vi "Audio.Play_Record.vi"(5 "volume":dbl=40.0 format="%#_13g", 6 "Record Device ID":u32, 7 "Play Device ID":u32=1, 8 "error in (no error)":errorcluster, 9 "RcdPostTime":dbl=0.05 format="%#_13g", 10 "RcdPreTime":dbl=0.05 format="%#_13g", 11 "Play Wvfrm":waveform(dbl)[](array[waveform])) -> (0 "Error Out":errorcluster, 2 "PlayDur(s)":dbl=1.0 format="%.2p", 3 "Rcd Wvfrm":waveform(dbl)[](array[waveform]))   [LabVIEW 2018]
uses:
  <vilib>/sound2/lvsound2.llb/Sampling Mode.ctl
  <vilib>/sound2/lvsound2.llb/Sound Data Format.ctl
  Utils/Errors/Error.Error Code List.ctl
  <vilib>/sound2/lvsound2.llb/Sound Output Set Volume (Single).vi
  <vilib>/sound2/lvsound2.llb/Sound Input Read (DBL).vi
  <vilib>/sound2/lvsound2.llb/Sound Output Write (DBL).vi
  <vilib>/KATE/Time/Time Utils.lvlib
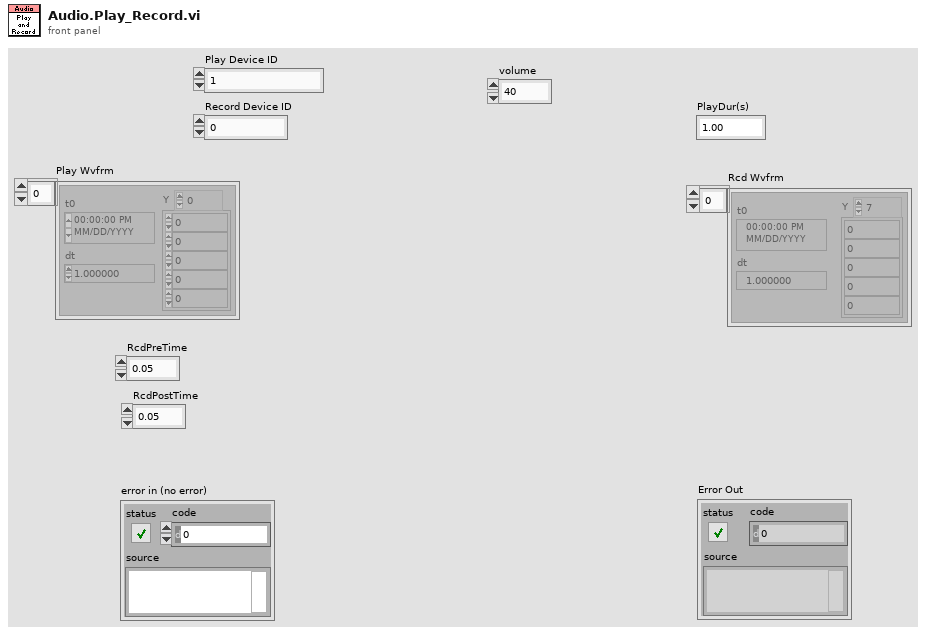
[diagram p1: front panel]
types:
  T1 = typedef "Sound Data Format.ctl" = cluster{"sample rate (S/s)":dbl, "number of channels":i32, "bits per sample":i32}
  T2 = typedef "Error.Error Code List.ctl" = i32
  T3 = typedef "Sampling Mode.ctl" = i32
  T4 = typedef "Sound Output Task ID.ctl" = u32
  T5 = typedef "Sound Input Task ID.ctl" = u32
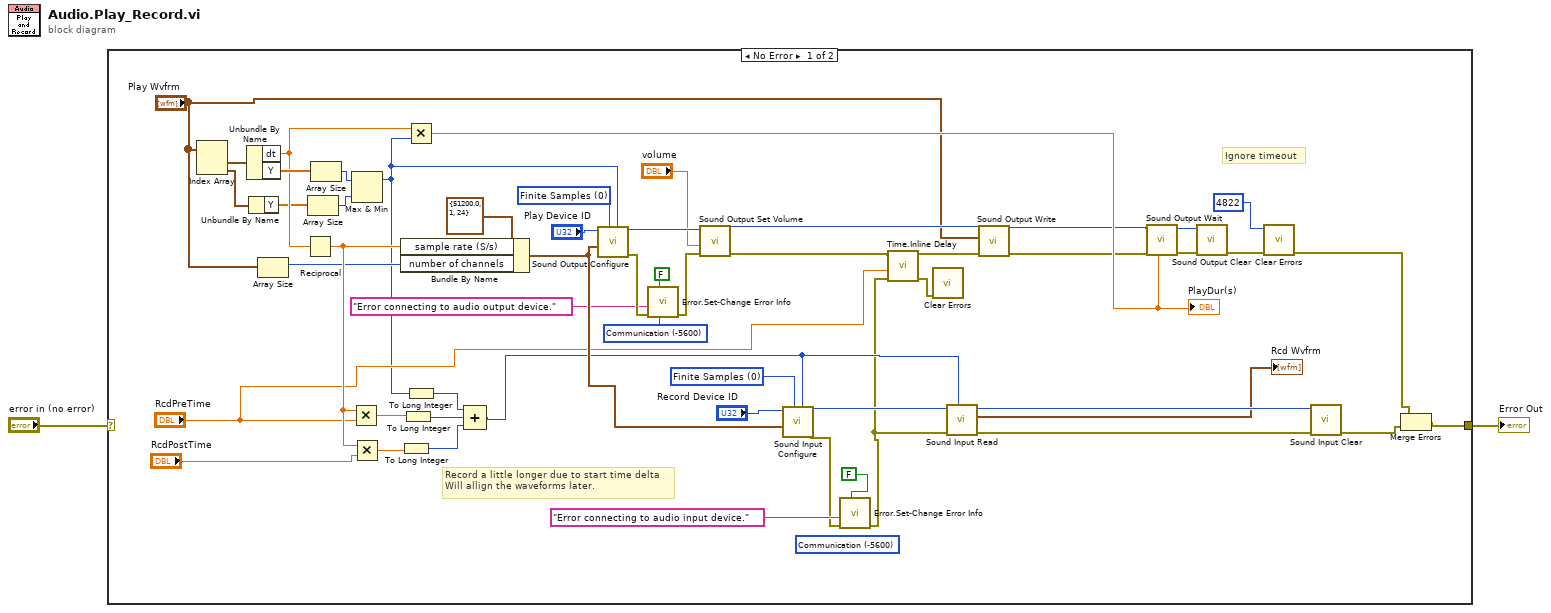
[diagram p0: block diagram]
diagram:
  n1 = case shown="No Error" "error in (no error)" {
    selector: "error in (no error)" -> [_ w57]
    tunnel: [w37 w57] -> w2
    frame No Error {
      (unwired) T2 -5600 items=["No Error"=0, "Abort"=-2, "Misc"=-5000, "Fixture Error"=-5100, "File IO - General"=-5200, "FIle IO - Config Error"=-5201, "Instrument - General"=-5300, "Instrument - Serial Com"=-5301, "Instrument - Camera"=-5302, "Instrument - PS"=-5303, "Instrument - Oscilloscope"=-5304, "Instrument - Function Gen"=-5305, "Instrument - Load"=-5306, "Instrument - Meter"=-5307, "Instrument - Power Control"=-5308, "Instrument - Motion"=-5309, "Instrument - RF"=-5310, "System Exe"=-5400, "Image Processing"=-5500, "Communication"=-5600, "Script - Syntax Error"=-6000, "Script - Invalid Name or Param"=-6100, "Script - Timeout"=-6200, "Invalid Data"=-6300, "FW Update Error"=-6500] ("Std Code")
      w34 = T2 -5600 items=["No Error"=0, "Abort"=-2, "Misc"=-5000, "Fixture Error"=-5100, "File IO - General"=-5200, "FIle IO - Config Error"=-5201, "Instrument - General"=-5300, "Instrument - Serial Com"=-5301, "Instrument - Camera"=-5302, "Instrument - PS"=-5303, "Instrument - Oscilloscope"=-5304, "Instrument - Function Gen"=-5305, "Instrument - Load"=-5306, "Instrument - Meter"=-5307, "Instrument - Power Control"=-5308, "Instrument - Motion"=-5309, "Instrument - RF"=-5310, "System Exe"=-5400, "Image Processing"=-5500, "Communication"=-5600, "Script - Syntax Error"=-6000, "Script - Invalid Name or Param"=-6100, "Script - Timeout"=-6200, "Invalid Data"=-6300, "FW Update Error"=-6500] ("Std Code")
      w51 = T3 0 items=["Finite Samples", "Continuous Samples"] ("sample mode")
      w53 = T3 0 items=["Finite Samples", "Continuous Samples"] ("sample mode")
      # "Ignore timeout"
      # "Record a little longer due to start time delta\nWill allign the waveforms later."
      n2 = Index Array(array="Play Wvfrm") -> (element #1=w28:waveform(dbl), element #2=w7:waveform(dbl))  [unwired: 2 in]
      n3 = Unbundle By Name(w28) -> ("dt"=w26:dbl, "Y"=w48:dbl[])
      n4 = Unbundle By Name(w7) -> ("Y"=w6:dbl[])
      n5 = Array Size(array="Play Wvfrm") -> (size(s)=w8:i32)
      n6 = Reciprocal(x=w26) -> (1/x=w25:dbl)
      n7 = Array Size(array=w6) -> (size(s)=w4:i32)
      n8 = Array Size(array=w48) -> (size(s)=w5:i32)
      n9 = Multiply(x=w25, y="RcdPreTime") -> (x*y=w47:dbl)
      n10 = Max & Min(x=w5, y=w4) -> (max(x,y)=w3:i32)  [unwired: 1 out]
      n11 = Multiply(x=w25, y="RcdPostTime") -> (x*y=w21:dbl)
      n12 = Bundle By Name(cluster=T1 {"sample rate (S/s)"=51200.0, "number of channels"=1, "bits per sample"=24} ("sound format"), "sample rate (S/s)"=w25, "number of channels"=w8) -> (w49:T1)
      n13 = To Long Integer(number=w21) -> (32bit integer=w20:i32)
      n14 = To Long Integer(number=w47) -> (32bit integer=w23:i32)
      n15 = Multiply(x=w26, y=w3) -> (x*y=w40:dbl)
      "PlayDur(s)" <- w40
      n16 = To Long Integer(number=w3) -> (32bit integer=w22:i32)
      n17 = Compound Arithmetic op=ADD(w22, w23, w20) -> (w19:i32)
      n18 = call <vilib>:"Sound Output Configure.vi"("number of samples/ch"=w3, "sample mode"=w53, "sound format"=w49, "device ID"="Play Device ID") -> ("error out"=w36:errorcluster, "task ID"=w56:T4)  [unwired: 6 in]
      n19 = call "Error.Set-Change Error Info.vi"("Std Code"=w34, "Append Details"=FALSE, "error in"=w36, "Description"="Error connecting to audio output device.") -> ("error out"=w35:errorcluster)  [unwired: 7 in]
      n20 = call-poly <vilib>:"Sound Output Set Volume.vi"("error in (no error)"=w35, "volume"="volume", "task ID"=w56) -> ("error out"=w14:errorcluster, "task ID out"=w17:T4)  [unwired: 7 in]
      n21 = call <vilib>:"Sound Input Configure.vi"("number of samples/ch"=w19, "sample mode"=w51, "sound format"=w49, "device ID"="Record Device ID") -> ("error out"=w31:errorcluster, "task ID"=w42:T5)  [unwired: 6 in]
      n22 = call "Error.Set-Change Error Info.vi"("Append Details"=FALSE, "error in"=w31, "Description"="Error connecting to audio input device.") -> ("error out"=w11:errorcluster)  [unwired: 8 in]
      n23 = call <vilib>:"Time.Inline Delay.vi"("error in (no error)"=w11, "Wait(secs)"="RcdPreTime", "error in top"=w14) -> ("error out"=w10:errorcluster, "error out top"=w13:errorcluster)  [unwired: 7 in]
      n24 = call <vilib>:"Clear Errors.vi"("error in (no error)"=w10) -> ()  [unwired: 5 in, 2 out]
      n25 = call-poly <vilib>:"Sound Input Read.vi"("number of samples/ch"=w19, "error in (no error)"=w11, "task ID"=w42) -> ("error out"=w18:errorcluster, "data"=→"Rcd Wvfrm":waveform(dbl)[], "task ID out"=w41:T5)  [unwired: 6 in]
      n26 = call-poly <vilib>:"Sound Output Write.vi"("error in (no error)"=w13, "data"="Play Wvfrm", "task ID"=w17) -> ("error out"=w15:errorcluster, "task ID out"=w16:T4)  [unwired: 7 in]
      n27 = call <vilib>:"Sound Output Wait.vi"("timeout (sec)"=w40, "error in (no error)"=w15, "task ID"=w16) -> ("error out"=w46:errorcluster, "task ID out"=w45:T4)  [unwired: 7 in]
      n28 = call <vilib>:"Sound Output Clear.vi"("error in (no error)"=w46, "task ID"=w45) -> ("error out"=w44:errorcluster)  [unwired: 9 in]
      n29 = call <vilib>:"Clear Errors.vi"("error in (no error)"=w44, "specific error code to clear (0: all)"=4822) -> ("error out"=w38:errorcluster)  [unwired: 4 in, 1 out]
      n30 = call <vilib>:"Sound Input Clear.vi"("error in (no error)"=w18, "task ID"=w41) -> ("error out"=w39:errorcluster)  [unwired: 9 in]
      n31 = Merge Errors(w38, w39) -> (w37:errorcluster)
    }
    frame Error {
    }
  }
  "Error Out" <- w2
